vi "ToolbarMenu.vi"(4 "Dim Transparency (90)":u8=90 max=99, 5 "Exit on VI Deactivation (T)":bool=TRUE, 6 "DimRegion (VI)":enum16{"VI", "Control", "Screen"}(ring), 7 "Caller Control Refnum":refnum<vi>, 8 "error in (no error)":errorcluster, 9 "ExitControls (Empty for all)":string[](array[string]), 10 "Position":T1, 11 "Menu Vi Reference":refnum<vi>) -> (0 "error out":errorcluster, 3 "ExitControl":cluster{"Name":string, "Value":variant})   [LabVIEW 2013, in "ToolbarMenu.lvlib"]
uses:
  ToolbarMenu.lvlib
  MenuPosition.ctl
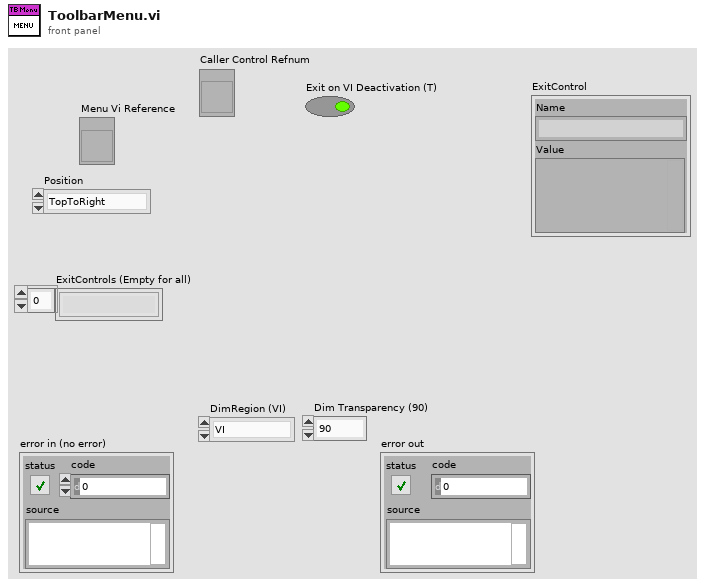
[diagram p1: front panel]
types:
  T1 = typedef "ToolbarMenu.lvlib/MenuPosition.ctl" = enum16{"TopToRight", "BottomToRight", "TopToLeft", "BottomToLeft"}
  T2 = enum32{"Invalid", "Standard", "Closed", "Hidden", "Minimized", "Maximized"}
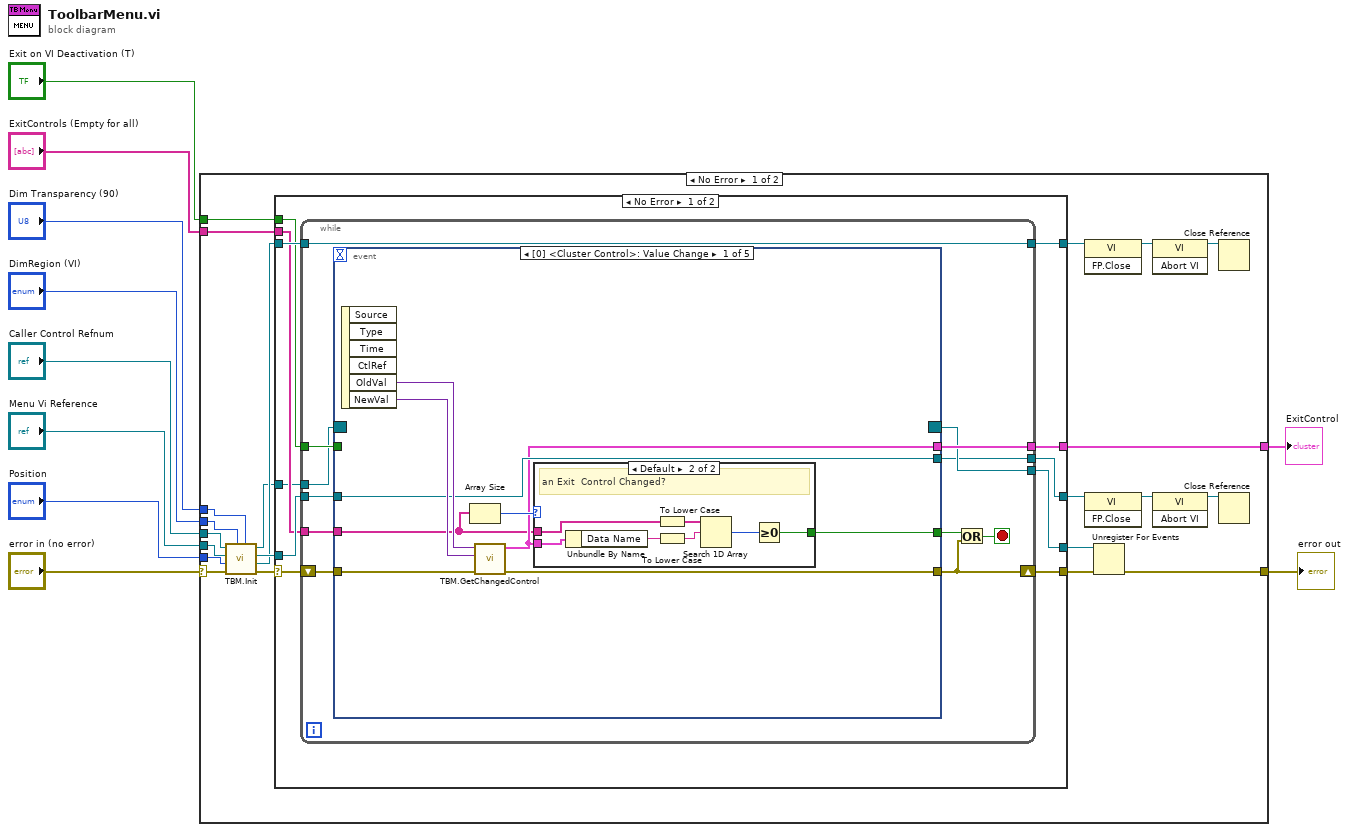
[diagram p0: block diagram]
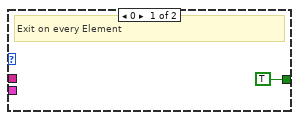
[diagram p2: hidden frame]
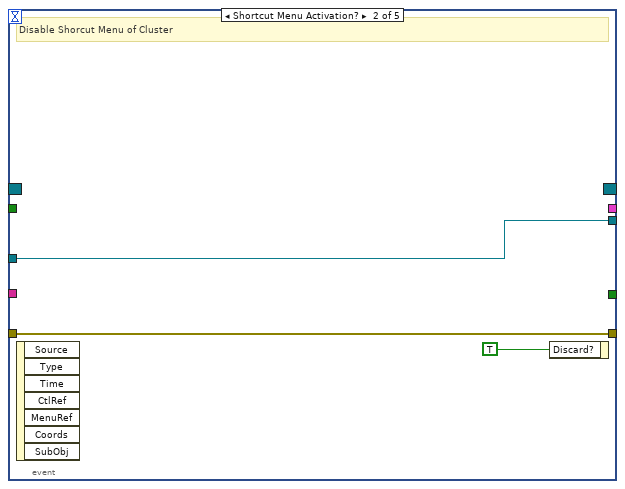
[diagram p3: hidden frame]
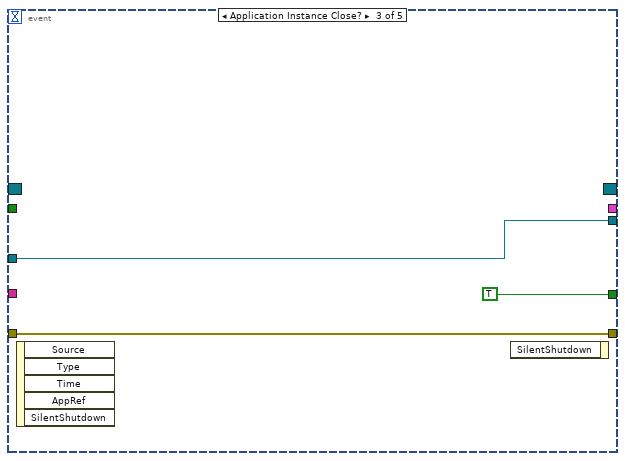
[diagram p4: hidden frame]
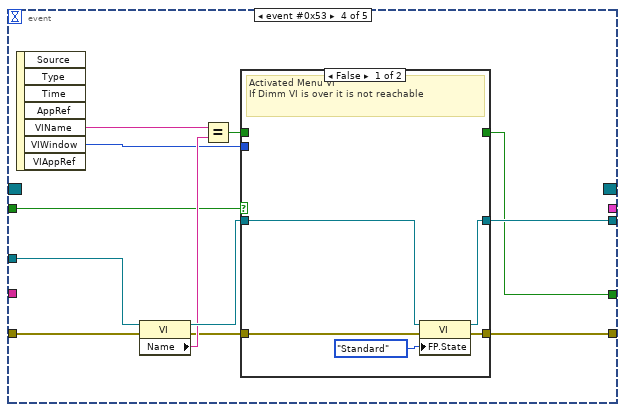
[diagram p5: hidden frame]
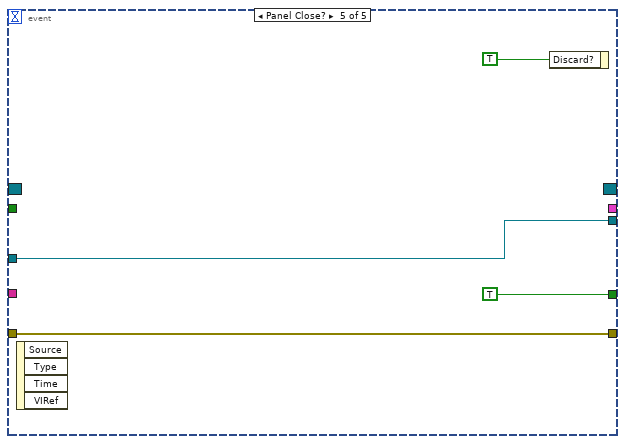
[diagram p7: hidden frame]
diagram:
  n1 = case shown="No Error" "error in (no error)" {
    selector: "error in (no error)" -> [w12 w107]
    tunnel: [w32 _] -> w10
    tunnel: "Caller Control Refnum" -> [w31 _]
    tunnel: "Menu Vi Reference" -> [w30 _]
    tunnel: "Position" -> [w29 _]
    tunnel: [w16 w107] -> w6
    tunnel: "Dim Transparency (90)" -> [w18 _]
    tunnel: "DimRegion (VI)" -> [w14 _]
    tunnel: "ExitControls (Empty for all)" -> [w17 _]
    tunnel: "Exit on VI Deactivation (T)" -> [w15 _]
    frame No Error {
      n2 = call "TBM.Init.vi"("Dim Transparency"=w18, "DimRegion"=w14, "error in (no error)"=w12, "Position"=w29, "Menu Vi Reference"=w30, "Control in"=w31) -> ("error out"=w11:errorcluster, "Dimmer reference"=w20:refnum<vi>, "Menu VI Refnum out"=w26:refnum<vi>, "Event Registration Refnum"=w13:refnum<event-registration>)  [unwired: 2 in]
      n3 = case shown="No Error" w11 {
        selector: w11 -> [w33 w106]
        tunnel: [w43 _] -> w32
        tunnel: [w42 w103] -> w28
        tunnel: [w41 w104] -> w27
        tunnel: w26 -> [w40 w103]
        tunnel: [w39 w106] -> w25
        tunnel: w20 -> [w38 w105]
        tunnel: [w37 w105] -> w19
        tunnel: w17 -> [w36 _]
        tunnel: w15 -> [w35 _]
        tunnel: w13 -> [w34 w104]
        frame No Error {
          n4 = while {
            tunnel: w40 -> [w51]
            tunnel: [w50] -> w42
            tunnel: [w55] -> w43
            shift-right: [w45] -> w39
            shift-left: w33 -> [w54]
            tunnel: [w52] -> w41
            tunnel: w38 -> [w44]
            tunnel: [w44] -> w37
            tunnel: w36 -> [w49]
            tunnel: w35 -> [w48]
            tunnel: w34 -> [w47]
            stop <- w53 stop-if-true
            n5 = event shown="[0] <Cluster Control>: Value Change" {
              selector: w47 -> [_ _ _ _ _]
              dyn-events: [_ _ _ _ _] -> w52
              timeout: _ -> [_ _ _ _ _]
              tunnel: [w64 _ TRUE w85 TRUE ("Discard?")] -> w46
              tunnel: [w57 _ _ _ _] -> w55
              tunnel: [w62 w74 w77 w84 w99] -> w45
              tunnel: w54 -> [w60 w74 w77 w89 w99]
              tunnel: w51 -> [w59 w73 w76 w90 w100]
              tunnel: [w59 w73 w76 w87 w100] -> w50
              tunnel: w49 -> [w56 _ _ _ _]
              tunnel: w48 -> [_ _ _ w80 _]
              event Value Change {
                n6 = event-data() -> ("OldVal"=w63:variant, "NewVal"=w61:variant)  [unwired: 1 in, 4 out]
                n7 = Array Size(array=w56) -> (size(s)=w58:i32)
                n8 = call "TBM.GetChangedControl.vi"("error in (no error)"=w60, "NewVal"=w61, "OldVal"=w63) -> ("error out"=w62:errorcluster, "Changed Control"=w57:cluster{"Data Name":string, "VElement":variant})  [unwired: 7 in]
                n9 = case shown="Default" w58 {
                  tunnel: [TRUE ("stop") w66] -> w64
                  tunnel: w57 -> [_ w72]
                  tunnel: w56 -> [_ w70]
                  frame 0 {
                    # "Exit on every Element"
                  }
                  frame Default {
                    # "an Exit  Control Changed?"
                    n10 = Unbundle By Name(w72) -> ("Data Name"=w71:string)
                    n11 = To Lower Case(string=w70) -> (all lower case string=w69:string[])
                    n12 = To Lower Case(string=w71) -> (all lower case string=w68:string)
                    n13 = Search 1D Array(1D array=w69, element=w68) -> (index of element=w67:i32)  [unwired: 1 in]
                    n14 = Greater Or Equal To 0?(x=w67) -> (x >= 0?=w66:bool)
                  }
                }
              }
              event Shortcut Menu Activation? {
                # "Disable Shorcut Menu of Cluster"
                n15 = event-data() -> ()  [unwired: 1 in, 7 out]
                n16 = event-data("Discard?"=TRUE) -> ()  [unwired: 1 in, 1 out]
              }
              event Application Instance Close? {
                n17 = event-data() -> ()  [unwired: 1 in, 5 out]
                n18 = event-data() -> ()  [unwired: 2 in, 1 out]
              }
              event event #0x53 {
                n19 = event-data() -> ("VIName"=w82:string, "VIWindow"=w79:i32)  [unwired: 1 in, 5 out]
                n20 = property class="VI"(reference=w90, error in=w89) -> (reference out=w88:refnum<vi>, error out=w81:errorcluster, "Name"=w83:string)
                n21 = Equal?(x=w82, y=w83) -> (x = y?=w86:bool)
                n22 = case shown="False" w80 {
                  tunnel: w88 -> [w95 w98]
                  tunnel: [w94 w98] -> w87
                  tunnel: w86 -> [_ w97]
                  tunnel: [_ w97] -> w85
                  tunnel: w81 -> [w91 w96]
                  tunnel: [w93 w96] -> w84
                  tunnel: w79 -> [_ _]
                  frame False {
                    # "Activated Menu VI\nIf Dimm VI is over it is not reachable"
                    n23 = property class="VI"(reference=w95, error in=w91, "FP.State"=T2."Standard" ("Front Panel Window:State")) -> (reference out=w94:refnum<vi>, error out=w93:errorcluster)
                  }
                  frame True {
                  }
                }
              }
              event Panel Close? {
                n24 = event-data() -> ()  [unwired: 1 in, 4 out]
                n25 = event-data("Discard?"=TRUE) -> ()  [unwired: 1 in, 1 out]
              }
            }
            n26 = Or(x=w46, y=w45) -> (x .or. y?=w53:bool)
          }
        }
        frame Error {
        }
      }
      n27 = invoke class="VI" method="FP.Close"(reference=w19) -> (reference out=w22:refnum<vi>)  [unwired: 2 in, 2 out]
      n28 = invoke class="VI" method="FP.Close"(reference=w28) -> (reference out=w24:refnum<vi>)  [unwired: 2 in, 2 out]
      n29 = Unregister For Events(event registration refnum=w27, error in=w25) -> (error out=w16:errorcluster)
      n30 = invoke class="VI" method="Abort VI"(reference=w22) -> (reference out=w21:refnum<vi>)  [unwired: 2 in, 2 out]
      n31 = invoke class="VI" method="Abort VI"(reference=w24) -> (reference out=w23:refnum<vi>)  [unwired: 2 in, 2 out]
      n32 = Close Reference(reference=w21) -> ()  [unwired: 1 in, 1 out]
      n33 = Close Reference(reference=w23) -> ()  [unwired: 1 in, 1 out]
    }
    frame Error {
    }
  }
  "ExitControl" <- w10
  "error out" <- w6
